vi "未命名 1.vi"() -> ()   [LabVIEW 2012]
panel:
  out "结果字符串":string
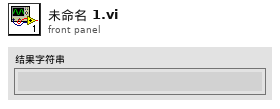
[diagram p1: front panel]
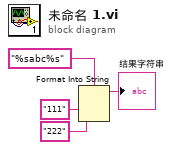
[diagram p0: block diagram]
diagram:
  n1 = Format Into String(format string="%sabc%s" ("格式字符串"), "111" ("输入 1"), "222" ("输入 2")) -> (resulting string=→"结果字符串":string)  [unwired: 2 in, 1 out]
